vi "留样信息存储.vi"() -> ()   [LabVIEW 2016, in "超标留样集成.lvlib"]
uses:
  DR803M4/Vis/Global variable/input variable.vi
  DR803M4/DR803M4.lvlib
panel:
  out "data输出":T1
  out "数组":string[](array[string])
  out "电子表格字符串":string
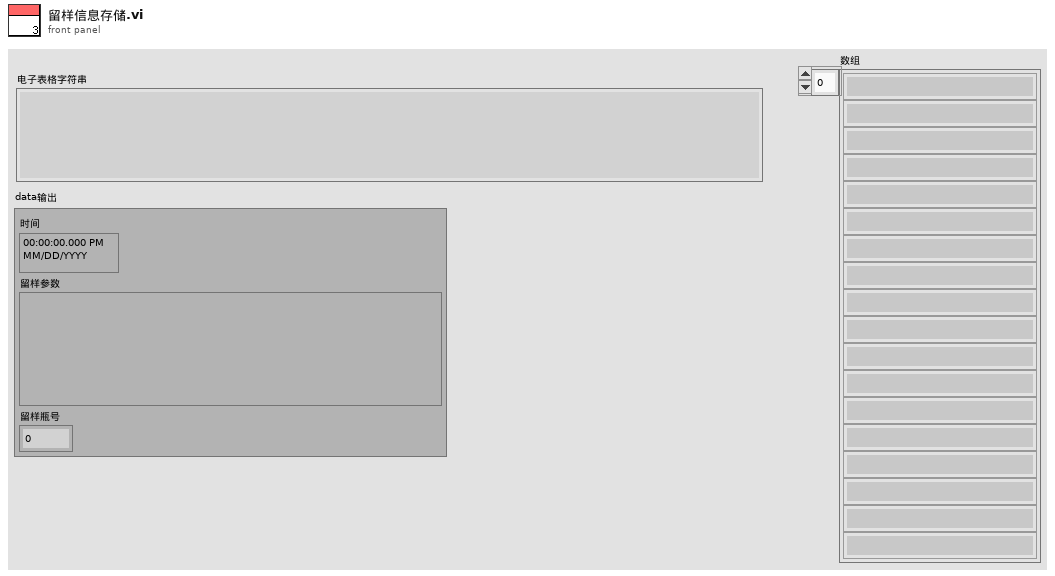
[diagram p1: front panel]
types:
  T1 = cluster{"时间":timestamp, "留样参数":string, "留样瓶号":dbl}
  T2 = typedef "报警信息字段定义.ctl" = cluster{"时间":timestamp, "参数":string, "元器件":string, "故障现象":string, "故障分析":string, "state":string, "code":string, "platform_alarm_code":string, "是否上报":string}
  T3 = enum16{"德润DR803M", "德润DR803L", "德润DR803F", "科盛超标留样", "德润DR803M4", "ESTD1200"}
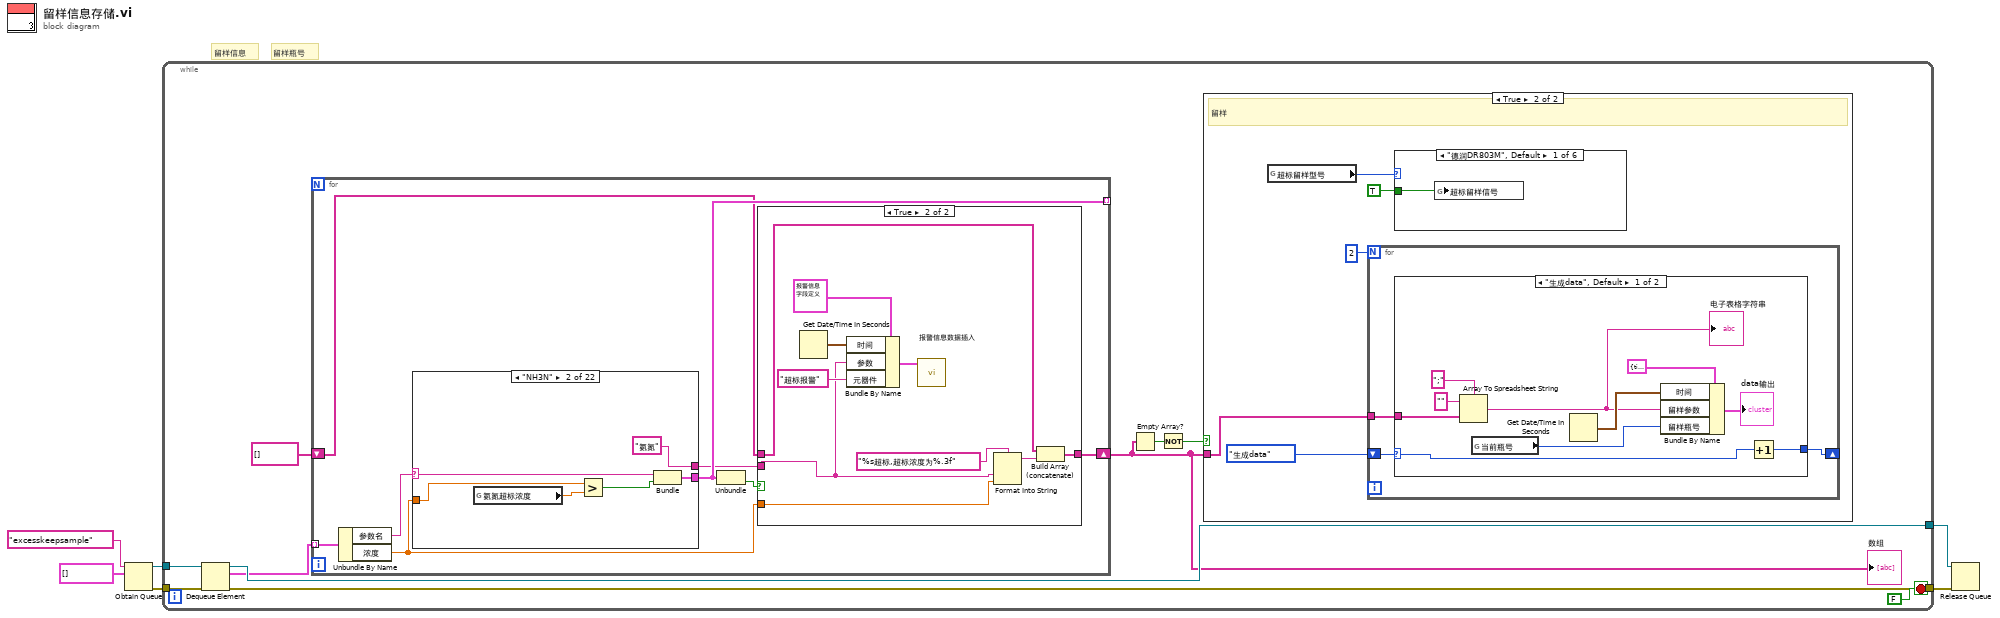
[diagram p0: block diagram]
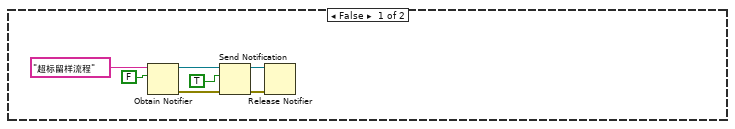
[diagram p2: hidden frame]
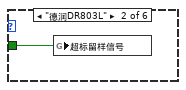
[diagram p3: hidden frame]
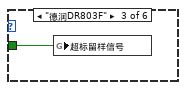
[diagram p4: hidden frame]
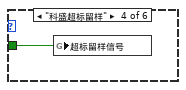
[diagram p5: hidden frame]
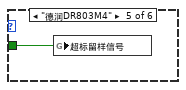
[diagram p6: hidden frame]
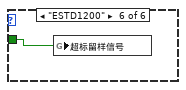
[diagram p7: hidden frame]
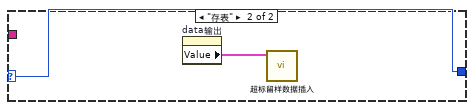
[diagram p8: hidden frame]
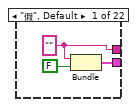
[diagram p10: hidden frame]
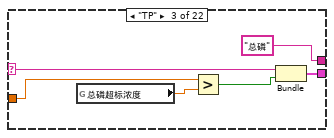
[diagram p11: hidden frame]
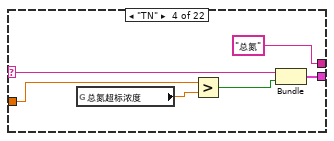
[diagram p12: hidden frame]
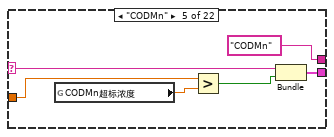
[diagram p13: hidden frame]
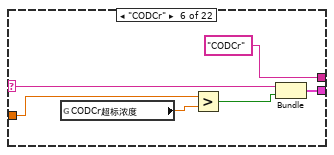
[diagram p14: hidden frame]
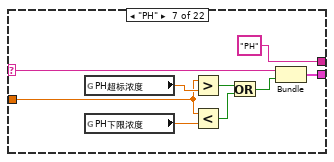
[diagram p15: hidden frame]
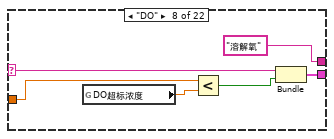
[diagram p16: hidden frame]
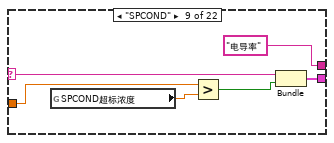
[diagram p17: hidden frame]
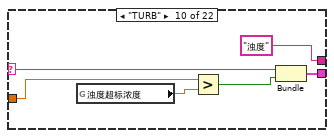
[diagram p18: hidden frame]
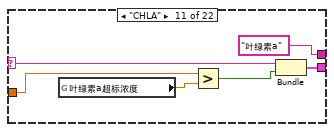
[diagram p19: hidden frame]
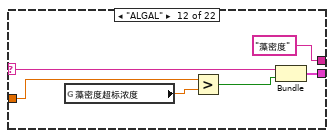
[diagram p20: hidden frame]
diagram:
  # "留样信息"
  # "留样瓶号"
  n1 = Obtain Queue(name (unnamed)="excesskeepsample" ("名称（未命名）"), element data type=cluster{"参数名":string, "浓度":dbl}[] []) -> (queue out=w4:refnum<queue>, error out=w3:errorcluster)  [unwired: 3 in, 1 out]
  n2 = while {
    tunnel: w4 -> [w16]
    tunnel: w3 -> [w14]
    tunnel: [w13] -> w2
    tunnel: [w12] -> w1
    stop <- FALSE stop-if-true
    n3 = Dequeue Element(queue=w16, error in (no error)=w14) -> (queue out=w13:refnum<queue>, element=w11:cluster{"参数名":string, "浓度":dbl}[], error out=w12:errorcluster)  [unwired: 1 in, 1 out]
    n4 = for {
      tunnel: w11 -> [w57] mode=indexing
      tunnel: [w54] -> _ mode=indexing
      shift-right: [w52] -> w9
      shift-left: string[] [] -> [w51]
      n5 = Unbundle By Name(w57) -> ("参数名"=w56:string, "浓度"=w55:dbl)
      n6 = case shown="\"NH3N\"" w56 {
        selector: w56 -> [_ w76 w81 w87 w94 w100 w110 w115 w121 w127 w133 w139 w145 w151 w156 w162 w168 w174 w180 w186 w192 w198]
        tunnel: w55 -> [_ w77 w82 w88 w95 w101 w107 w116 w122 w128 w134 w140 w146 w152 w155 w161 w167 w173 w179 w185 w191 w197]
        tunnel: [w70 w74 w80 w86 w93 w99 w109 w114 w120 w126 w132 w138 w144 w150 w158 w164 w170 w176 w182 w188 w194 w200] -> w54
        tunnel: [w69 "氨氮" "总磷" "总氮" "CODMn" "CODCr" "PH" "溶解氧" "电导率" "浊度" "叶绿素a" "藻密度" "蓝绿藻" "ORP" "COD" "铅" "镉" "铜" "锌" "镍" "锰" "汞"] -> w50
        frame "假", Default {
          w69 = ""
          n7 = Bundle(w69, FALSE) -> (w70:cluster{string, bool})  [unwired: 1 in]
        }
        frame "NH3N" {
          n8 = global read "断电保存全局.vi" "氨氮超标浓度"() -> (w73:dbl)
          n9 = Greater?(x=w77, y=w73) -> (0:w75:bool)
          n10 = Bundle(w76, w75) -> (w74:cluster{string, bool})  [unwired: 1 in]
        }
        frame "TP" {
          n11 = global read "断电保存全局.vi" "总磷超标浓度"() -> (w79:dbl)
          n12 = Greater?(x=w82, y=w79) -> (0:w83:bool)
          n13 = Bundle(w81, w83) -> (w80:cluster{string, bool})  [unwired: 1 in]
        }
        frame "TN" {
          n14 = global read "断电保存全局.vi" "总氮超标浓度"() -> (w85:dbl)
          n15 = Greater?(x=w88, y=w85) -> (0:w89:bool)
          n16 = Bundle(w87, w89) -> (w86:cluster{string, bool})  [unwired: 1 in]
        }
        frame "CODMn" {
          n17 = global read "断电保存全局.vi" "CODMn超标浓度"() -> (w91:dbl)
          n18 = Greater?(x=w95, y=w91) -> (0:w92:bool)
          n19 = Bundle(w94, w92) -> (w93:cluster{string, bool})  [unwired: 1 in]
        }
        frame "CODCr" {
          n20 = global read "断电保存全局.vi" "CODCr超标浓度"() -> (w97:dbl)
          n21 = Greater?(x=w101, y=w97) -> (0:w98:bool)
          n22 = Bundle(w100, w98) -> (w99:cluster{string, bool})  [unwired: 1 in]
        }
        frame "PH" {
          n23 = global read "断电保存全局.vi" "PH超标浓度"() -> (w108:dbl)
          n24 = global read "断电保存全局.vi" "PH下限浓度"() -> (w106:dbl)
          n25 = Greater?(x=w107, y=w108) -> (0:w105:bool)
          n26 = Less?(x=w107, y=w106) -> (x < y?=w104:bool)
          n27 = Or(x=w105, y=w104) -> (x .or. y?=w103:bool)
          n28 = Bundle(w110, w103) -> (w109:cluster{string, bool})  [unwired: 1 in]
        }
        frame "DO" {
          n29 = global read "断电保存全局.vi" "DO超标浓度"() -> (w112:dbl)
          n30 = Less?(x=w116, y=w112) -> (x < y?=w113:bool)
          n31 = Bundle(w115, w113) -> (w114:cluster{string, bool})  [unwired: 1 in]
        }
        frame "SPCOND" {
          n32 = global read "断电保存全局.vi" "SPCOND超标浓度"() -> (w118:dbl)
          n33 = Greater?(x=w122, y=w118) -> (0:w119:bool)
          n34 = Bundle(w121, w119) -> (w120:cluster{string, bool})  [unwired: 1 in]
        }
        frame "TURB" {
          n35 = global read "断电保存全局.vi" "浊度超标浓度"() -> (w124:dbl)
          n36 = Greater?(x=w128, y=w124) -> (0:w125:bool)
          n37 = Bundle(w127, w125) -> (w126:cluster{string, bool})  [unwired: 1 in]
        }
        frame "CHLA" {
          n38 = global read "断电保存全局.vi" "叶绿素a超标浓度"() -> (w130:dbl)
          n39 = Greater?(x=w134, y=w130) -> (0:w131:bool)
          n40 = Bundle(w133, w131) -> (w132:cluster{string, bool})  [unwired: 1 in]
        }
        frame "ALGAL" {
          n41 = global read "断电保存全局.vi" "藻密度超标浓度"() -> (w136:dbl)
          n42 = Greater?(x=w140, y=w136) -> (0:w137:bool)
          n43 = Bundle(w139, w137) -> (w138:cluster{string, bool})  [unwired: 1 in]
        }
        frame "Cyanobacteria" {
          n44 = global read "断电保存全局.vi" "蓝绿藻超标浓度"() -> (w142:dbl)
          n45 = Greater?(x=w146, y=w142) -> (0:w143:bool)
          n46 = Bundle(w145, w143) -> (w144:cluster{string, bool})  [unwired: 1 in]
        }
        frame "ORP" {
          n47 = global read "断电保存全局.vi" "ORP超标浓度"() -> (w148:dbl)
          n48 = Greater?(x=w152, y=w148) -> (0:w149:bool)
          n49 = Bundle(w151, w149) -> (w150:cluster{string, bool})  [unwired: 1 in]
        }
        frame "COD" {
          n50 = global read "断电保存全局.vi" "COD超标浓度"() -> (w154:dbl)
          n51 = Greater?(x=w155, y=w154) -> (0:w157:bool)
          n52 = Bundle(w156, w157) -> (w158:cluster{string, bool})  [unwired: 1 in]
        }
        frame "PB" {
          n53 = global read "断电保存全局.vi" "铅超标浓度"() -> (w160:dbl)
          n54 = Greater?(x=w161, y=w160) -> (0:w163:bool)
          n55 = Bundle(w162, w163) -> (w164:cluster{string, bool})  [unwired: 1 in]
        }
        frame "CD" {
          n56 = global read "断电保存全局.vi" "镉超标浓度"() -> (w166:dbl)
          n57 = Greater?(x=w167, y=w166) -> (0:w169:bool)
          n58 = Bundle(w168, w169) -> (w170:cluster{string, bool})  [unwired: 1 in]
        }
        frame "CU" {
          n59 = global read "断电保存全局.vi" "铜超标浓度"() -> (w172:dbl)
          n60 = Greater?(x=w173, y=w172) -> (0:w175:bool)
          n61 = Bundle(w174, w175) -> (w176:cluster{string, bool})  [unwired: 1 in]
        }
        frame "ZN" {
          n62 = global read "断电保存全局.vi" "锌超标浓度"() -> (w178:dbl)
          n63 = Greater?(x=w179, y=w178) -> (0:w181:bool)
          n64 = Bundle(w180, w181) -> (w182:cluster{string, bool})  [unwired: 1 in]
        }
        frame "NI" {
          n65 = global read "断电保存全局.vi" "镍超标浓度"() -> (w184:dbl)
          n66 = Greater?(x=w185, y=w184) -> (0:w187:bool)
          n67 = Bundle(w186, w187) -> (w188:cluster{string, bool})  [unwired: 1 in]
        }
        frame "MN" {
          n68 = global read "断电保存全局.vi" "锰超标浓度"() -> (w190:dbl)
          n69 = Greater?(x=w191, y=w190) -> (0:w193:bool)
          n70 = Bundle(w192, w193) -> (w194:cluster{string, bool})  [unwired: 1 in]
        }
        frame "HG" {
          n71 = global read "断电保存全局.vi" "汞超标浓度"() -> (w196:dbl)
          n72 = Greater?(x=w197, y=w196) -> (0:w199:bool)
          n73 = Bundle(w198, w199) -> (w200:cluster{string, bool})  [unwired: 1 in]
        }
      }
      n74 = Unbundle(w54) -> (w53:bool)  [unwired: 1 out]
      n75 = case shown="True" w53 {
        tunnel: w55 -> [_ w68]
        tunnel: [w58 w64] -> w52
        tunnel: w51 -> [w58 w66]
        tunnel: w50 -> [_ w59]
        frame False {
        }
        frame True {
          n76 = Get Date/Time In Seconds() -> (seconds since 1Jan1904=w61:timestamp)
          n77 = Bundle By Name(cluster=T2 {"时间"=timestamp(0 s since 1904-01-01), "参数"="水样测试", "元器件"="N", "故障现象"="", "故障分析"="", "state"="", "code"="", "platform_alarm_code"="", "是否上报"=""} ("data"), "时间"=w61, "参数"=w59, "元器件"="超标报警" ("报警信息")) -> (w62:T2)
          n78 = call "报警信息数据插入.vi"("data"=w62) -> ()  [unwired: 9 in, 1 out]
          n79 = Format Into String(format string="%s超标,超标浓度为%.3f" ("格式字符串"), w59, w68) -> (resulting string=w65:string)  [unwired: 2 in, 1 out]
          n80 = Build Array (concatenate)(w66, w65) -> (w64:string[])
        }
      }
    }
    "数组" <- w9
    n81 = Empty Array?(array=w9) -> (empty?=w8:bool)
    n82 = Not(x=w8) -> (.not. x?=w7:bool)
    n83 = case shown="True" w7 {
      tunnel: w9 -> [_ w26]
      frame False {
        n84 = Obtain Notifier(name (unnamed)="超标留样流程" ("名称（未命名）"), notification data type=FALSE ("采样完成")) -> (notifier out=w21:refnum<notifier>, error out=w20:errorcluster)  [unwired: 2 in, 1 out]
        n85 = Send Notification(notification=TRUE ("通知"), notifier=w21, error in (no error)=w20) -> (notifier out=w19:refnum<notifier>, error out=w18:errorcluster)
        n86 = Release Notifier(notifier=w19, error in (no error)=w18) -> ()  [unwired: 1 in, 3 out]
      }
      frame True {
        # "留样"
        n87 = global read "断电保存全局.vi" "超标留样型号"() -> (w25:T3)
        n88 = for {
          N: 2 -> [_]
          tunnel: w26 -> [w36]
          shift-right: [w35] -> _
          shift-left: enum16{"生成data", "存表"}."生成data" -> [w37]
          n89 = case shown="\"生成data\", Default" w37 {
            selector: w37 -> [w44 w49]
            tunnel: w36 -> [w45 _]
            tunnel: [w43 w49] -> w35
            frame "生成data", Default {
              n90 = Array To Spreadsheet String(delimiter (Tab)=";" ("分隔符(Tab)"), array=w45, 3:"") -> (spreadsheet string=w41:string)
              "电子表格字符串" <- w41
              n91 = global read "外部交互全局.vi" "当前瓶号"() -> (w38:u16)
              n92 = Get Date/Time In Seconds() -> (seconds since 1Jan1904=w47:timestamp)
              n93 = Bundle By Name(cluster=T1 {"时间"=timestamp(3687928779.282504 s since 1904-01-01), "留样参数"="NH3N超标,超标浓度为0.000\r\n留样瓶号:0", "留样瓶号"=0.0} ("data输出"), "时间"=w47, "留样参数"=w41, "留样瓶号"=w38) -> (→"data输出":T1)
              n94 = Increment(x=w44) -> (x+1=w43:enum16{"生成data", "存表"})
            }
            frame "存表" {
              n95 = property on="data输出" class="Clust (strict)"() -> ("Value"=w48:T1)  [unwired: 2 in, 2 out]
              n96 = call "超标留样数据插入.vi"("data输出"=w48) -> ()  [unwired: 9 in, 1 out]
            }
          }
        }
        n97 = case shown="\"德润DR803M\", Default" w25 {
          tunnel: TRUE ("超标留样信号") -> [w29 w30 w31 w32 w33 w34]
          frame "德润DR803M", Default {
            n98 = global write "超标留样全局.vi" "超标留样信号"(w29) -> ()
          }
          frame "德润DR803L" {
            n99 = global write "串口参数断电保存全局变量.vi" "超标留样信号"(w30) -> ()
          }
          frame "德润DR803F" {
            n100 = global write "超标留样全局.vi" "超标留样信号"(w31) -> ()
          }
          frame "科盛超标留样" {
            n101 = global write "超标留样全局.vi" "超标留样信号"(w32) -> ()
          }
          frame "德润DR803M4" {
            n102 = global write "input variable.vi" "超标留样信号"(w33) -> ()
          }
          frame "ESTD1200" {
            n103 = global write "串口参数断电保存全局变量.vi" "超标留样信号"(w34) -> ()
          }
        }
      }
    }
  }
  n104 = Release Queue(queue=w2, error in (no error)=w1) -> ()  [unwired: 1 in, 3 out]
